vi "纳清蓝绿藻电极校准.vi"() -> ()   [LabVIEW 2016, in "斯坦道多参数.lvlib"]
uses:
  <vilib>/Utility/miscctls.llb/LVPointTypeDef.ctl
  <vilib>/Utility/miscctls.llb/LVPositionTypeDef.ctl
  <vilib>/Analysis/NI_AALBase.lvlib
panel:
  out "通讯状态":string
  out "温度校准参数":sgl
  out "第三点校准值":dbl
  out "标液3":sgl
  out "第二点校准值":dbl
  out "第一点校准值":dbl
  in  "校准停止":bool
  in  "校准启动":bool
  in  "校准模式":enum16{"两点校准", "单点校准", "三点校准"}(ring)=enum."单点校准"
  out "最小值":sgl format="%#.2f"
  out "最大值":sgl format="%#.2f"
  out "波形图表":u16(graph) caption="历史曲线"
  out "mean":dbl caption="均值" format="%#.2f"
  out "standard deviation":dbl caption="标准差" format="%#.2f"
  out "变异系数":dbl format="%#.6f"
  out "测量值":sgl
  out "提示":string
  out "标液2":sgl
  out "标液1":sgl
  out "原始光强数值":u16 caption="信号值"
  out "温度":dbl
  # "藻密度电极设定"
  # "℃"
  # "ug/L"
  # "℃"
  # "请选择校准模式:"
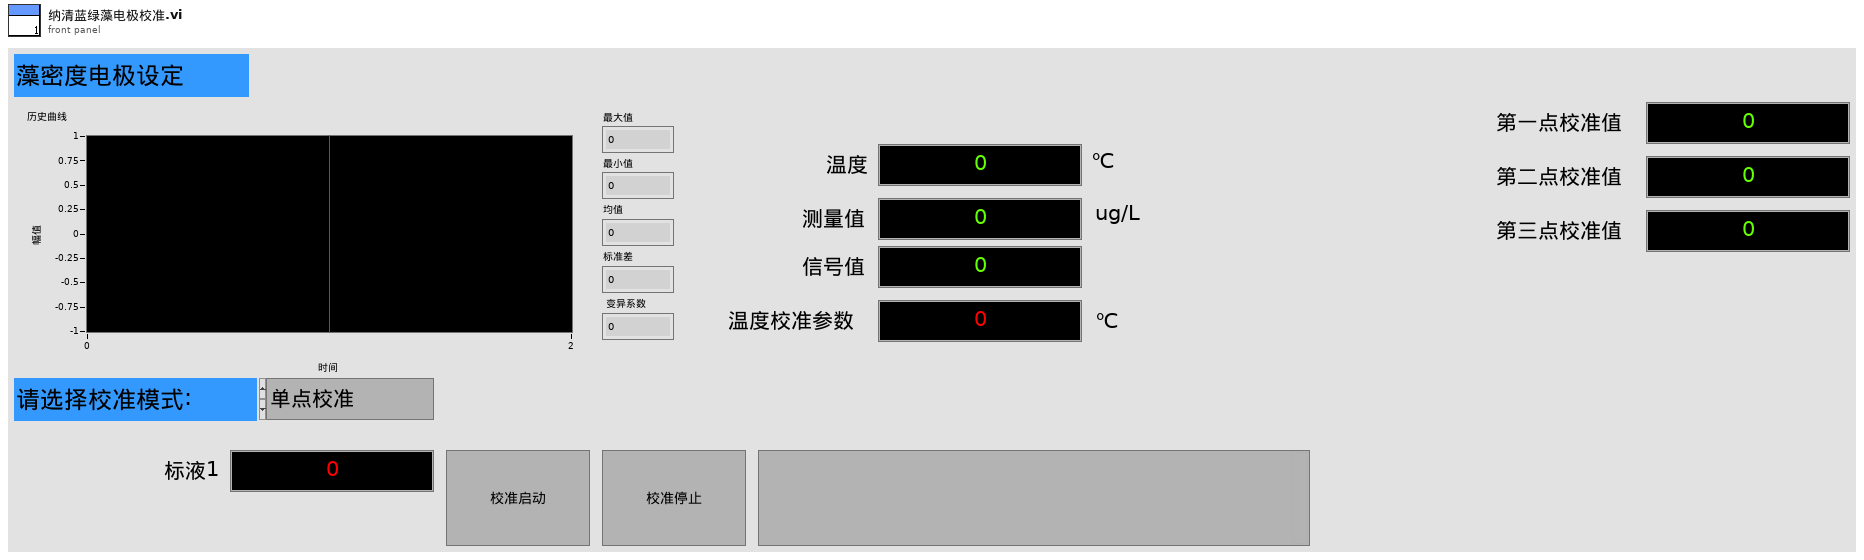
[diagram p1: front panel]
types:
  T1 = typedef "LVPointTypeDef.ctl" = cluster{"Horizontal":i16, "Vertical":i16}
  T2 = typedef "斯坦道多参数.lvlib/校准步骤.ctl" = enum16{"待机", "放置第一点标液", "第一点校准启动", "第一点校准写入", "第一点校准失败", "放置第二点标液", "第二点校准启动", "第二点校准写入", "第二点校准失败", "放置第三点标液", "第三点校准启动", "第三点校准写入", "第三点校准失败", "校准结果写入", "校准结束"}
  T3 = cluster{"报警码":u16, "蓝绿藻":sgl, "温度数据":sgl, "原始光强数值":u16, "0X0006_NC":u16, "平均次数":u16, "清扫模式":u16, "清扫次数":u16, "清扫间隔分钟":u16, "0X000B_NC":string, "产品名称":string, "序列号":string, "硬件版本":string, "软件版本":string, "通讯地址":u16, "波特率":u16, "设备类型":u16, "0X0026_NC":string, "0X0030_NC":u16, "第一点原始光强":u16, "第一点校准数据":sgl, "第二点原始光强":u16, "第二点校准数据":sgl, "第三点原始光强":u16, "第三点校准数据":sgl, "探头校准命令":u16, "温度校准参数":sgl, "温度校准命令":u16}
  T4 = typedef "LVPositionTypeDef.ctl" = cluster{"Left":i32, "Top":i32}
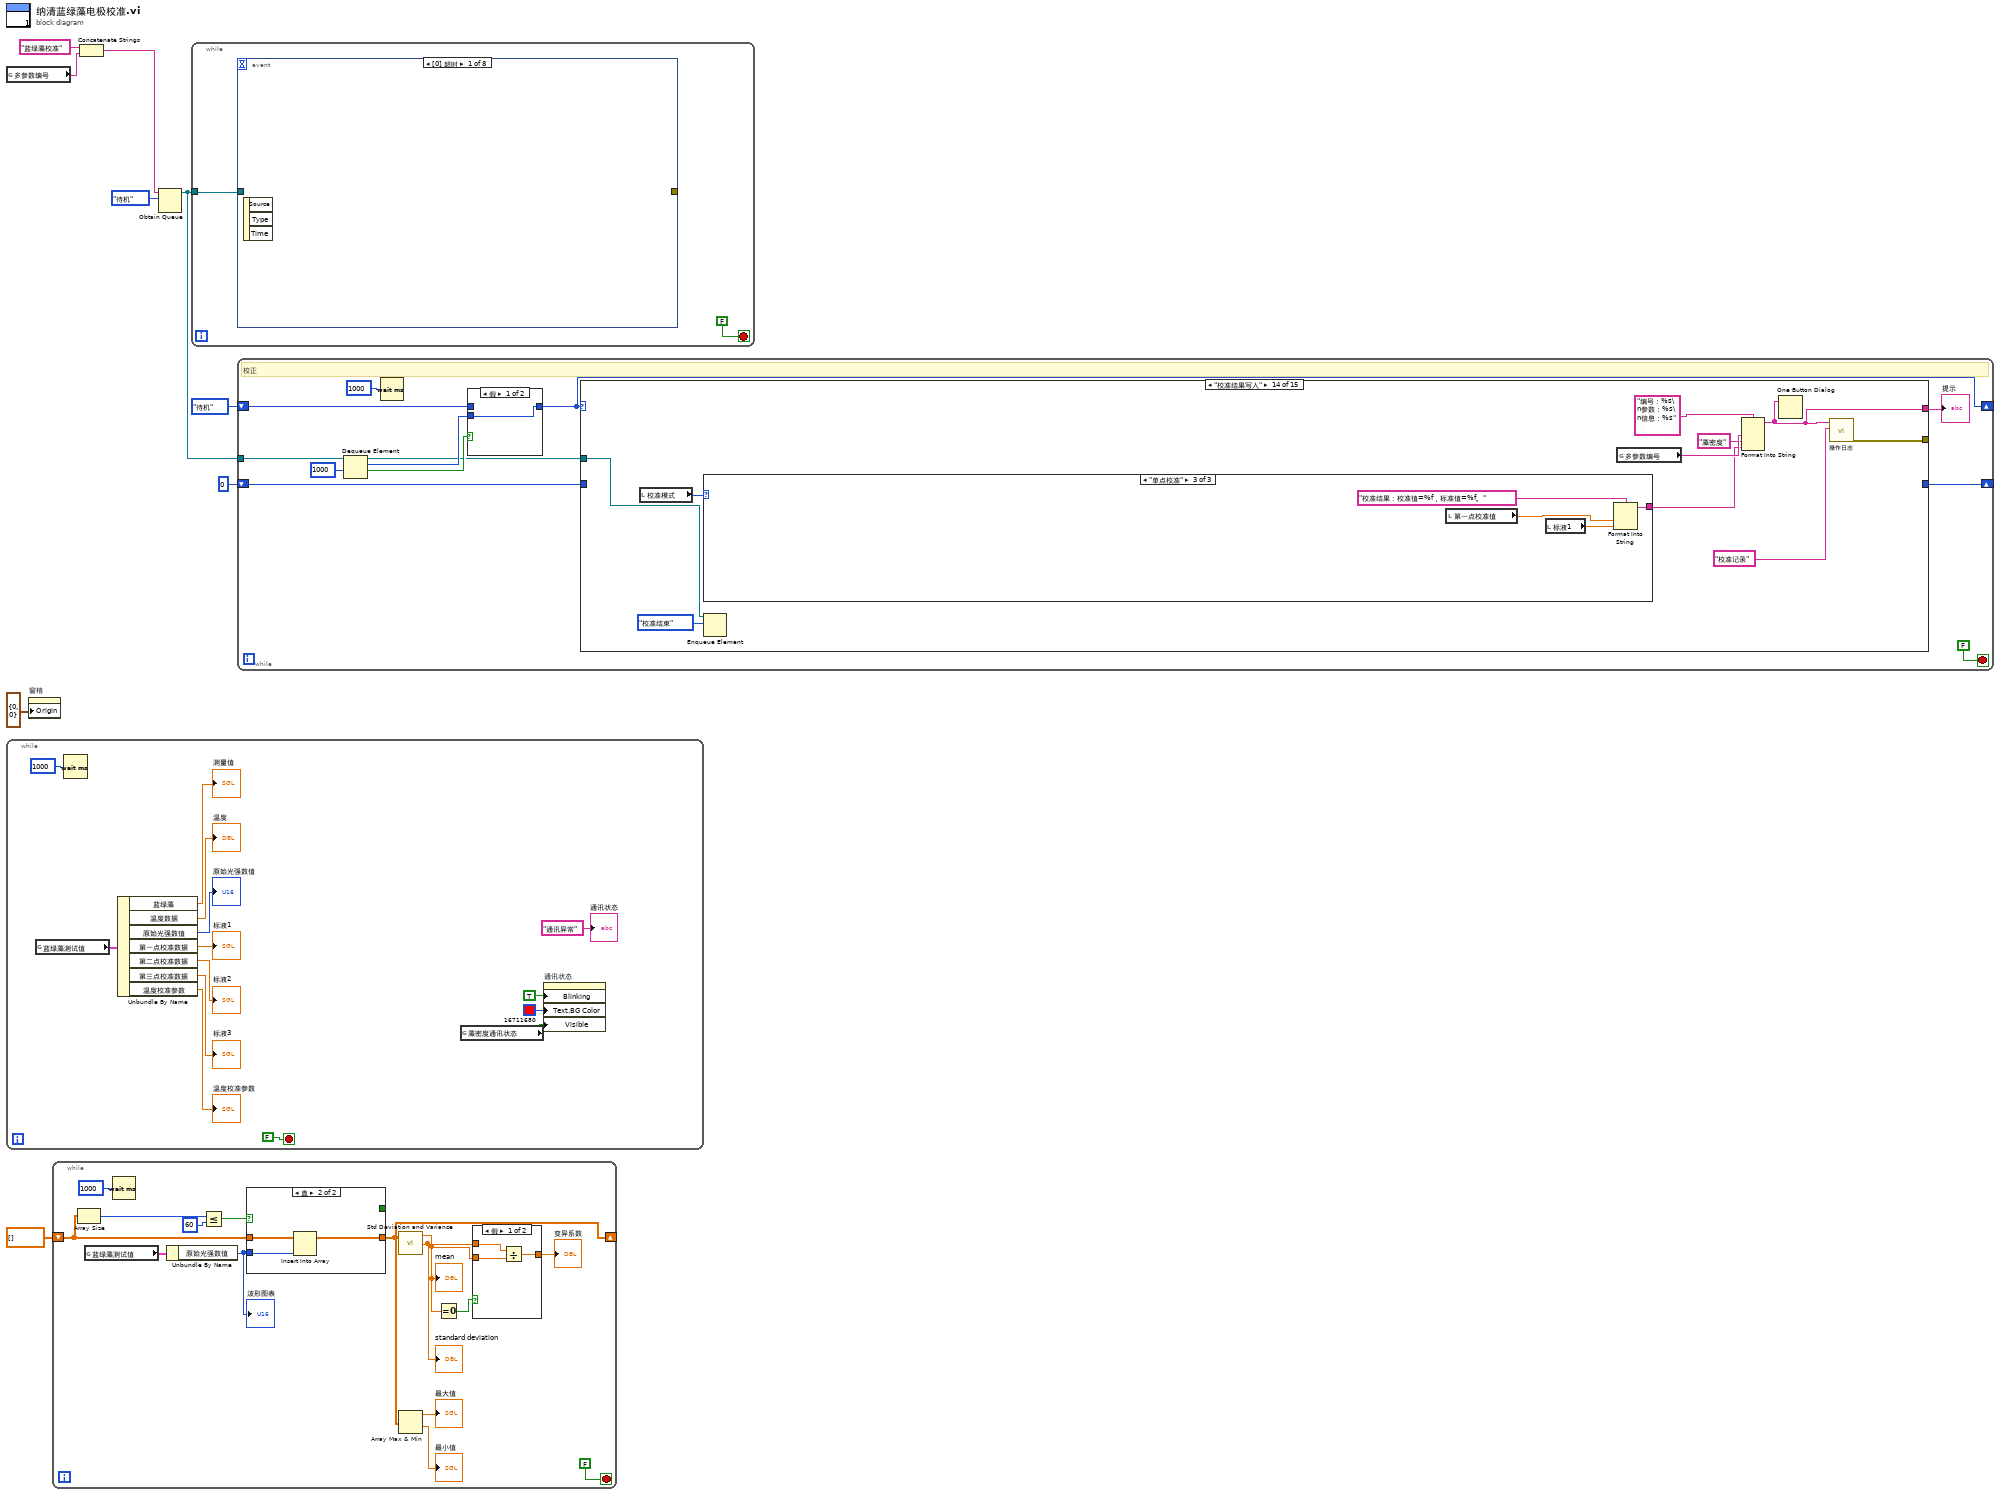
[diagram p0: block diagram]
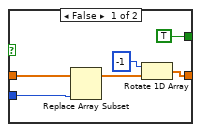
[diagram p3: hidden frame]
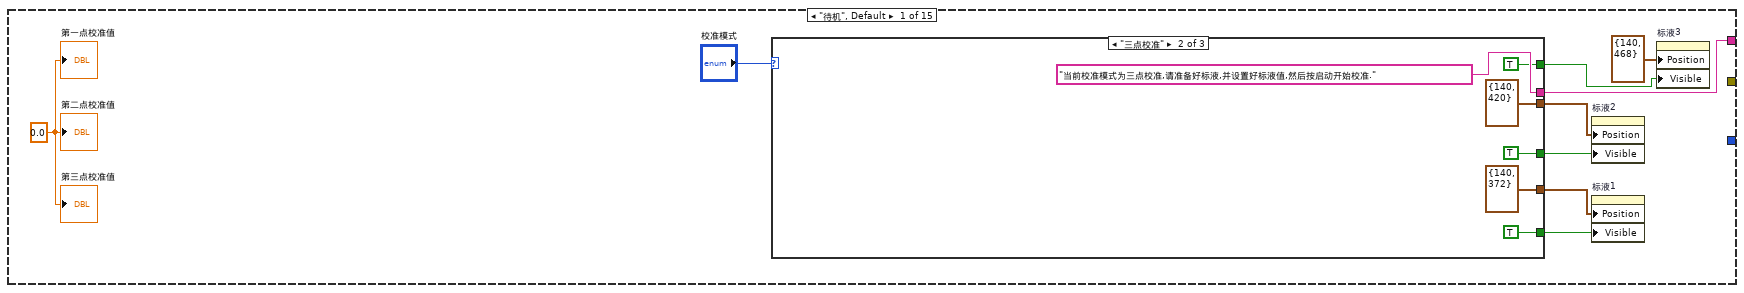
[diagram p5: hidden frame]
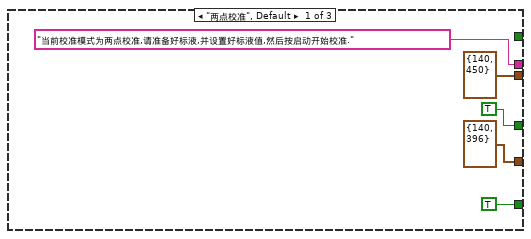
[diagram p6: hidden frame]
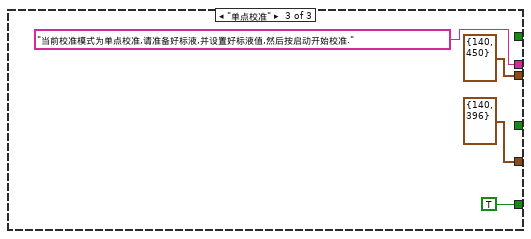
[diagram p7: hidden frame]
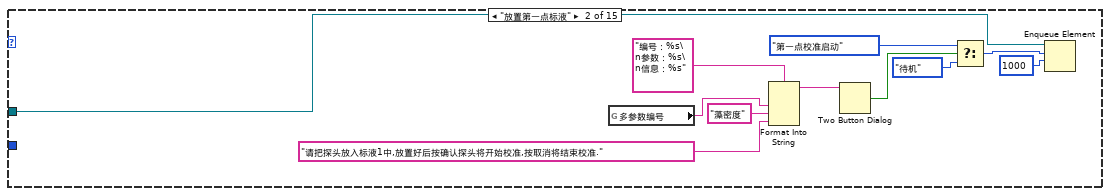
[diagram p8: hidden frame]
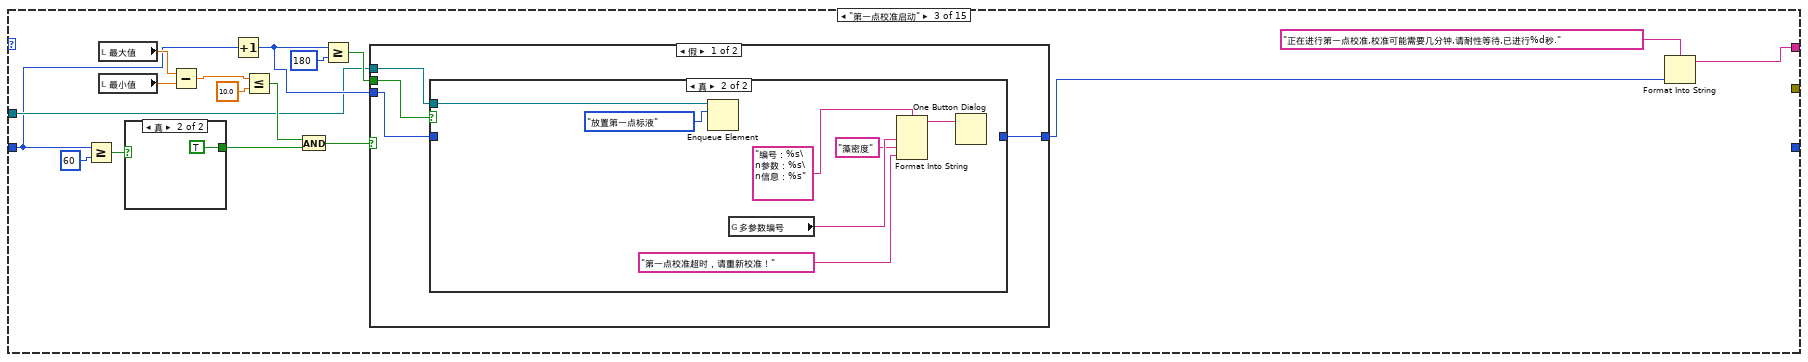
[diagram p9: hidden frame]
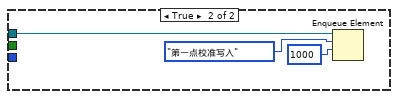
[diagram p11: hidden frame]
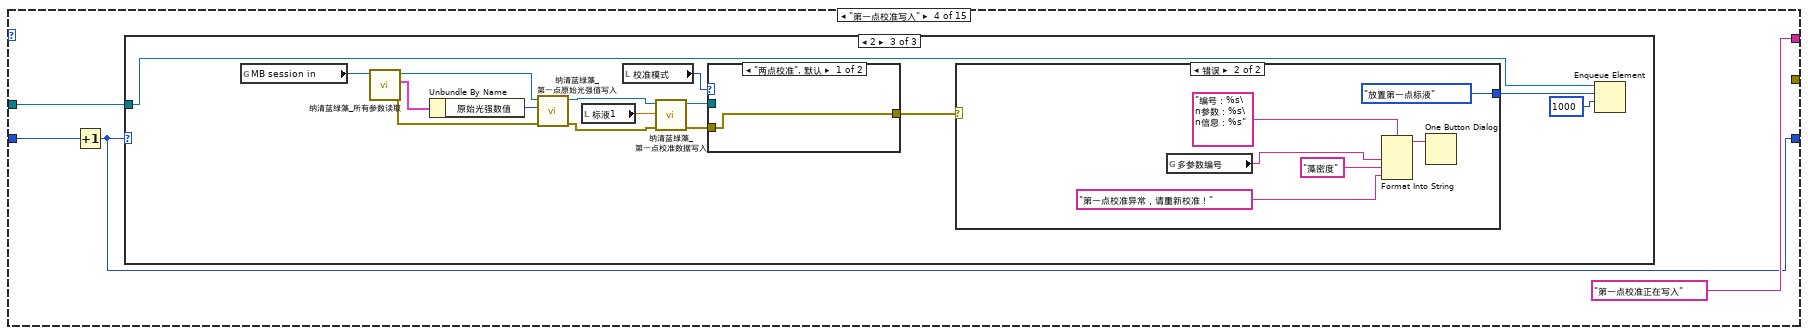
[diagram p13: hidden frame]
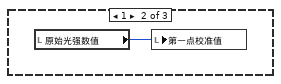
[diagram p15: hidden frame]
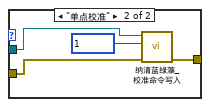
[diagram p16: hidden frame]
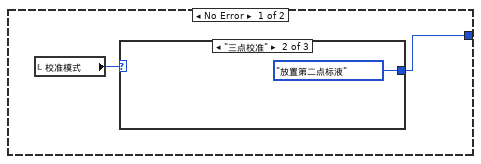
[diagram p17: hidden frame]
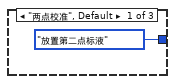
[diagram p18: hidden frame]
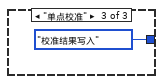
[diagram p19: hidden frame]
diagram:
  n1 = global read "多参数全局变量.vi" "多参数编号"() -> (w1:string)
  n2 = while {
    stop <- FALSE stop-if-true
    n3 = global read "纳清过程全局变量.vi" "蓝绿藻测试值"() -> (w21:T3)
    n4 = Wait (ms)(milliseconds to wait=u32 1000 ("等待时间（毫秒）")) -> ()  [unwired: 1 out]
    n5 = Unbundle By Name(w21) -> ("蓝绿藻"=→"测量值":sgl, "温度数据"=→"温度":sgl, "原始光强数值"=→"原始光强数值":u16, "第一点校准数据"=→"标液1":sgl, "第二点校准数据"=→"标液2":sgl, "第三点校准数据"=→"标液3":sgl, "温度校准参数"=→"温度校准参数":sgl)
    n6 = global read "多参数全局变量.vi" "藻密度通讯状态"() -> (w10:bool)
    n7 = property on="通讯状态" class="Str"("Blinking"=TRUE ("闪烁"), "Text.BG Color"=u32 16711680, "Visible"=w10) -> ()  [unwired: 2 in, 2 out]
    "通讯状态" <- "通讯异常" ("当前串口")
  }
  n8 = property on="窗格" class="Pane"("Origin"=T1 {"Horizontal"=0, "Vertical"=0} ("原点")) -> ()  [unwired: 2 in, 2 out]
  n9 = while {
    shift-right: [w28] -> _
    shift-left: sgl[] [] -> [w34]
    stop <- FALSE stop-if-true
    n10 = Array Size(array=w34) -> (size(s)=w36:i32)
    n11 = global read "纳清过程全局变量.vi" "蓝绿藻测试值"() -> (w24:T3)
    n12 = Wait (ms)(milliseconds to wait=u32 1000 ("等待时间（毫秒）")) -> ()  [unwired: 1 out]
    n13 = Unbundle By Name(w24) -> ("原始光强数值"=w25:u16)
    "波形图表" <- w25
    n14 = Less Or Equal?(x=w36, y=60) -> (x <= y?=w35:bool)
    n15 = case shown="真" w35 {
      tunnel: w34 -> [w47 w50]
      tunnel: w25 -> [w45 w49]
      tunnel: [w43 w48] -> w28
      tunnel: [TRUE _] -> _
      frame False {
        n16 = Replace Array Subset(array=w47, new element=w45) -> (w46:sgl[])  [unwired: 1 in]
        n17 = Rotate 1D Array(1:w46, 2:-1 ("n")) -> (0:w43:sgl[])
      }
      frame True {
        n18 = Insert Into Array(array=w50, new element=w49) -> (w48:sgl[])  [unwired: 1 in]
      }
    }
    n19 = call <vilib>:"Std Deviation and Variance.vi"("X"=w28) -> ("mean"=w32:dbl, "standard deviation"=w31:dbl)  [unwired: 1 in, 1 out]
    "mean" <- w32
    "standard deviation" <- w31
    n20 = Array Max & Min(array=w28) -> (max value=→"最大值":sgl, min value=→"最小值":sgl)  [unwired: 2 out]
    n21 = Equal To 0?(x=w32) -> (x = 0?=w33:bool)
    n22 = case shown="假" w33 {
      tunnel: w31 -> [w41 _]
      tunnel: [w40 _] -> w30
      tunnel: w32 -> [w39 _]
      frame False {
        n23 = Divide(x=w41, y=w39) -> (x/y=w40:dbl)
      }
      frame True {
      }
    }
    "变异系数" <- w30
  }
  n24 = Concatenate Strings("蓝绿藻校准" ("名称（未命名）"), w1) -> (w2:string)
  n25 = Obtain Queue(name (unnamed)=w2, element data type=校准步骤."待机" ("枚举")) -> (queue out=w4:refnum<queue>)  [unwired: 3 in, 2 out]
  n26 = while {
    tunnel: w4 -> [w51]
    stop <- FALSE stop-if-true
    n27 = event shown="[0] 超时" {
      selector: _ -> [_ _ _ _ _ _ _ _]
      dyn-events: _ -> [_ _ _ _ _ _ _ _]
      timeout: _ -> [_ _ _ _ _ _ _ _]
      tunnel: [_ _ w58 w62 w65 w66 _ _] -> _
      tunnel: w51 -> [_ _ _ _ _ _ w73 w75]
      event Timeout {
        n28 = event-data() -> ()  [unwired: 1 in, 3 out]
      }
      event "标液1", "标液2", "标液3", "温度校准参数": Mouse Down {
        n29 = event-data() -> ("CtlRef"=w53:refnum<vi>)  [unwired: 1 in, 7 out]
        n30 = property class="DigNum (严格)"(reference=w53) -> (reference out=w54:refnum<vi>, "Value"=w55:sgl)  [unwired: 1 in, 1 out]
        n31 = call "数字键盘.vi"("OldNumber"=w55) -> ("NewNumber"=w56:dbl)  [unwired: 1 in]
        n32 = property class="DigNum (严格)"(reference=w54, "Val(Sgnl)"=w56) -> ()  [unwired: 1 in, 2 out]
      }
      event "标液1": Value Change {
        n33 = event-data() -> ("NewVal"=w57:sgl)  [unwired: 1 in, 5 out]
        n34 = global read "多参数全局变量.vi" "MB session in"() -> (w59:refnum<class "MB_Master.lvclass">)
        n35 = call "纳清蓝绿藻_第一点校准数据写入.vi"("数值"=w57, "MB session in"=w59) -> ("error out"=w58:errorcluster)  [unwired: 8 in, 1 out]
      }
      event "标液2": Value Change {
        n36 = event-data() -> ("NewVal"=w61:sgl)  [unwired: 1 in, 5 out]
        n37 = global read "多参数全局变量.vi" "MB session in"() -> (w60:refnum<class "MB_Master.lvclass">)
        n38 = call "纳清蓝绿藻_第二点校准数据写入.vi"("数值"=w61, "MB session in"=w60) -> ("error out"=w62:errorcluster)  [unwired: 8 in, 1 out]
      }
      event "标液3": Value Change {
        n39 = event-data() -> ("NewVal"=w63:sgl)  [unwired: 1 in, 5 out]
        n40 = global read "多参数全局变量.vi" "MB session in"() -> (w64:refnum<class "MB_Master.lvclass">)
        n41 = call "纳清蓝绿藻_第三点校准数据写入.vi"("数值"=w63, "MB session in"=w64) -> ("error out"=w65:errorcluster)  [unwired: 8 in, 1 out]
      }
      event "温度校准参数": Value Change {
        n42 = event-data() -> ("NewVal"=w71:sgl)  [unwired: 1 in, 5 out]
        n43 = global read "多参数全局变量.vi" "MB session in"() -> (w70:refnum<class "MB_Master.lvclass">)
        n44 = call "纳清蓝绿藻_温度校准参数写入.vi"("数值"=w71, "MB session in"=w70) -> ("error out"=w72:errorcluster, "MB session out"=w69:refnum<class "MB_Master.lvclass">)  [unwired: 8 in]
        n45 = call "纳清蓝绿藻_温度校准命令写入.vi"("error in (no error)"=w72, "数值"=u16 1 ("starting address"), "MB session in"=w69) -> ("error out"=w67:errorcluster)  [unwired: 7 in, 1 out]
        n46 = call <vilib>:"Simple Error Handler.vi"("error in (no error)"=w67) -> ("error out"=w66:errorcluster)  [unwired: 4 in, 4 out]
      }
      event "校准启动": Value Change {
        n47 = event-data() -> ()  [unwired: 1 in, 6 out]
        n48 = Enqueue Element(queue=w73, element=校准步骤."放置第一点标液" ("元素")) -> ()  [unwired: 2 in, 3 out]
      }
      event "校准停止": Value Change {
        n49 = event-data() -> ()  [unwired: 1 in, 6 out]
        n50 = Flush Queue(queue=w75) -> (queue out=w76:refnum<queue>)  [unwired: 1 in, 2 out]
        n51 = Enqueue Element(queue=w76, element=校准步骤."待机" ("元素"), timeout in ms (-1)=1000 ("超时毫秒(-1)")) -> ()  [unwired: 1 in, 3 out]
      }
    }
  }
  n52 = while "While循环" {
    shift-right: [w80] -> _
    shift-left: 校准步骤."待机" ("枚举") -> [w82]
    shift-right: [w79] -> _
    shift-left: 0 -> [w88]
    tunnel: w4 -> [w83]
    stop <- FALSE stop-if-true
    # "校正"
    n53 = Dequeue Element(queue=w83, timeout in ms (-1)=1000 ("超时毫秒(-1)")) -> (queue out=w81:refnum<queue>, element=w84:T2, timed out?=w85:bool)  [unwired: 1 in, 1 out]
    n54 = Wait (ms)(milliseconds to wait=u32 1000 ("等待时间（毫秒）")) -> ()  [unwired: 1 out]
    n55 = case shown="假" w85 {
      tunnel: w84 -> [w91 _]
      tunnel: [w91 w92] -> w80
      tunnel: w82 -> [_ w92]
      frame False {
      }
      frame True {
      }
    }
    n56 = case shown="\"校准结果写入\"" w80 {
      tunnel: [w100 _ w128 "第一点校准正在写入" ("提示") _ _ w210 "第二点校准正在写入" ("提示") "第二点校准失败" ("提示") _ "第三点校准正在写入" ("提示") w322 "第三点校准失败" ("提示") w355 w382] -> w87
      tunnel: w88 -> [_ _ w130 w163 _ _ w211 w243 _ _ w291 w323 _ _ _]
      tunnel: [_ _ _ w161 _ _ w209 w241 _ _ w289 w321 _ _ _] -> w79
      tunnel: w81 -> [_ w123 w131 w162 _ w202 w212 w242 _ w283 w290 w324 _ w362 _]
      tunnel: [_ _ _ _ _ _ _ _ _ _ _ _ _ w360 _] -> _
      frame "待机", Default {
        w93 = 0.0 ("第一点校准值")
        n57 = case shown="\"三点校准\"" "校准模式" {
          tunnel: ["当前校准模式为两点校准,请准备好标液,并设置好标液值,然后按启动开始校准." ("提示") "当前校准模式为三点校准,请准备好标液,并设置好标液值,然后按启动开始校准." ("提示") "当前校准模式为单点校准,请准备好标液,并设置好标液值,然后按启动开始校准." ("提示")] -> w100
          tunnel: [TRUE ("可见") TRUE ("可见") _] -> w96
          tunnel: [T4 {"Left"=140, "Top"=396} ("位置") T4 {"Left"=140, "Top"=372} ("位置") T4 {"Left"=140, "Top"=396} ("位置")] -> w99
          tunnel: [T4 {"Left"=140, "Top"=450} ("位置 2") T4 {"Left"=140, "Top"=420} ("位置 2") T4 {"Left"=140, "Top"=450} ("位置 2")] -> w98
          tunnel: [_ TRUE ("可见") _] -> w95
          tunnel: [TRUE ("可见") TRUE ("可见") TRUE ("可见")] -> w94
          frame "两点校准", Default {
          }
          frame "三点校准" {
          }
          frame "单点校准" {
          }
        }
        n58 = property on="标液2" class="DigNum (严格)"("Position"=w98, "Visible"=w96) -> ()  [unwired: 2 in, 2 out]
        n59 = property on="标液1" class="DigNum (严格)"("Position"=w99, "Visible"=w94) -> ()  [unwired: 2 in, 2 out]
        n60 = property on="标液3" class="DigNum (严格)"("Position"=T4 {"Left"=140, "Top"=468} ("位置 3"), "Visible"=w95) -> ()  [unwired: 2 in, 2 out]
        "第一点校准值" <- w93
        "第二点校准值" <- w93
        "第三点校准值" <- w93
      }
      frame "放置第一点标液" {
        n61 = global read "多参数全局变量.vi" "多参数编号"() -> (w121:string)
        n62 = Format Into String(format string="编号：%s\n参数：%s\n信息：%s" ("格式字符串"), w121, "藻密度" ("输入 2"), "请把探头放入标液1中,放置好后按确认探头将开始校准,按取消将结束校准." ("消息")) -> (resulting string=w119:string)  [unwired: 2 in, 1 out]
        n63 = Two Button Dialog(message=w119) -> (T button?=w117:bool)  [unwired: 2 in]
        n64 = Select(t=校准步骤."第一点校准启动" ("元素"), s=w117, f=校准步骤."待机" ("元素")) -> (s? t:f=w124:T2)
        n65 = Enqueue Element(queue=w123, element=w124, timeout in ms (-1)=1000 ("超时毫秒(-1)")) -> ()  [unwired: 1 in, 3 out]
      }
      frame "第一点校准启动" {
        n66 = Greater Or Equal?(x=w130, y=60) -> (x >= y?=w137:bool)
        n67 = local read "最大值"() -> (w140:sgl)
        n68 = local read "最小值"() -> (w139:sgl)
        n69 = case shown="真" w137 {
          tunnel: [_ TRUE] -> w138
          frame False {
          }
          frame True {
          }
        }
        n70 = Subtract(x=w140, y=w139) -> (x-y=w141:sgl)
        n71 = Increment(x=w130) -> (x+1=w144:i32)
        n72 = Less Or Equal?(x=w141, y=10.0) -> (x <= y?=w134:bool)
        n73 = And(x=w134, y=w138) -> (x .and. y?=w142:bool)
        n74 = Greater Or Equal?(x=w144, y=180) -> (x >= y?=w143:bool)
        n75 = case shown="假" w142 {
          tunnel: w131 -> [w147 w159]
          tunnel: w143 -> [w148 _]
          tunnel: w144 -> [w146 _]
          tunnel: [w145 _] -> w129
          frame False {
            n76 = case shown="真" w148 {
              tunnel: w147 -> [_ w156]
              tunnel: w146 -> [w149 _]
              tunnel: [w149 _] -> w145
              frame False {
              }
              frame True {
                n77 = Enqueue Element(queue=w156, element=校准步骤."放置第一点标液" ("元素")) -> ()  [unwired: 2 in, 3 out]
                n78 = global read "多参数全局变量.vi" "多参数编号"() -> (w153:string)
                n79 = Format Into String(format string="编号：%s\n参数：%s\n信息：%s" ("格式字符串"), w153, "藻密度" ("输入 2"), "第一点校准超时，请重新校准！" ("error source (\" \")")) -> (resulting string=w150:string)  [unwired: 2 in, 1 out]
                n80 = One Button Dialog(message=w150) -> ()  [unwired: 1 in, 1 out]
              }
            }
          }
          frame True {
            n81 = Enqueue Element(queue=w159, element=校准步骤."第一点校准写入" ("元素"), timeout in ms (-1)=1000 ("超时毫秒(-1)")) -> ()  [unwired: 1 in, 3 out]
          }
        }
        n82 = Format Into String(format string="正在进行第一点校准,校准可能需要几分钟,请耐性等待,已进行%d秒." ("格式字符串"), w129) -> (resulting string=w128:string)  [unwired: 2 in, 1 out]
      }
      frame "第一点校准写入" {
        n83 = Increment(x=w163) -> (x+1=w161:i32)
        n84 = case shown="2" w161 {
          tunnel: w162 -> [_ _ w180]
          frame 0, Default {
          }
          frame 1 {
            n85 = local read "原始光强数值"() -> (w165:u16)
            n86 = local write "第一点校准值"(w165) -> ()
          }
          frame 2 {
            n87 = global read "多参数全局变量.vi" "MB session in"() -> (w176:refnum<class "MB_Master.lvclass">)
            n88 = call "纳清蓝绿藻_所有参数读取.vi"("MB session in"=w176) -> ("error out"=w178:errorcluster, "输出值"=w175:T3, "MB session out"=w177:refnum<class "MB_Master.lvclass">)  [unwired: 8 in]
            n89 = Unbundle By Name(w175) -> ("原始光强数值"=w174:u16)
            n90 = call "纳清蓝绿藻_第一点原始光强值写入.vi"("error in (no error)"=w178, "数值"=w174, "MB session in"=w177) -> ("error out"=w173:errorcluster, "MB session out"=w172:refnum<class "MB_Master.lvclass">)  [unwired: 7 in]
            n91 = local read "标液1"() -> (w169:sgl)
            n92 = local read "校准模式"() -> (w166:enum16{"两点校准", "单点校准", "三点校准"})
            n93 = call "纳清蓝绿藻_第一点校准数据写入.vi"("error in (no error)"=w173, "数值"=w169, "MB session in"=w172) -> ("error out"=w171:errorcluster, "MB session out"=w170:refnum<class "MB_Master.lvclass">)  [unwired: 7 in]
            n94 = case shown="\"两点校准\", 默认" w166 {
              tunnel: w171 -> [w181 w185]
              tunnel: w170 -> [_ w184]
              tunnel: [w181 w182] -> w168
              frame "两点校准", Default {
              }
              frame "单点校准" {
                n95 = call "纳清蓝绿藻_校准命令写入.vi"("error in (no error)"=w185, "数值"=u16 1 ("starting address"), "MB session in"=w184) -> ("error out"=w182:errorcluster)  [unwired: 7 in, 1 out]
              }
            }
            n96 = case shown="错误" w168 {
              tunnel: [w186 校准步骤."放置第一点标液" ("元素")] -> w167
              frame No Error {
                n97 = local read "校准模式"() -> (w187:enum16{"两点校准", "单点校准", "三点校准"})
                n98 = case shown="\"三点校准\"" w187 {
                  tunnel: [校准步骤."放置第二点标液" ("元素") 校准步骤."放置第二点标液" ("元素") 校准步骤."校准结果写入" ("元素")] -> w186
                  frame "两点校准", Default {
                  }
                  frame "三点校准" {
                  }
                  frame "单点校准" {
                  }
                }
              }
              frame Error {
                n99 = global read "多参数全局变量.vi" "多参数编号"() -> (w195:string)
                n100 = Format Into String(format string="编号：%s\n参数：%s\n信息：%s" ("格式字符串"), w195, "藻密度" ("输入 2"), "第一点校准异常，请重新校准！" ("error source (\" \")")) -> (resulting string=w192:string)  [unwired: 2 in, 1 out]
                n101 = One Button Dialog(message=w192) -> ()  [unwired: 1 in, 1 out]
              }
            }
            n102 = Enqueue Element(queue=w180, element=w167, timeout in ms (-1)=1000 ("超时毫秒(-1)")) -> ()  [unwired: 1 in, 3 out]
          }
        }
      }
      frame "第一点校准失败" {
      }
      frame "放置第二点标液" {
        n103 = global read "多参数全局变量.vi" "多参数编号"() -> (w200:string)
        n104 = Format Into String(format string="编号：%s\n参数：%s\n信息：%s" ("格式字符串"), w200, "藻密度" ("输入 2"), "请把探头放入标液2中,放置好后按确认将继续校准,按取消将结束校准." ("消息")) -> (resulting string=w198:string)  [unwired: 2 in, 1 out]
        n105 = Two Button Dialog(message=w198) -> (T button?=w206:bool)  [unwired: 2 in]
        n106 = Select(t=校准步骤."第二点校准启动" ("元素"), s=w206, f=校准步骤."待机" ("元素")) -> (s? t:f=w203:T2)
        n107 = Enqueue Element(queue=w202, element=w203, timeout in ms (-1)=1000 ("超时毫秒(-1)")) -> ()  [unwired: 1 in, 3 out]
      }
      frame "第二点校准启动" {
        n108 = Greater Or Equal?(x=w211, y=60) -> (x >= y?=w217:bool)
        n109 = local read "最大值"() -> (w220:sgl)
        n110 = local read "最小值"() -> (w219:sgl)
        n111 = case shown="真" w217 {
          tunnel: [_ TRUE] -> w218
          frame False {
          }
          frame True {
          }
        }
        n112 = Subtract(x=w220, y=w219) -> (x-y=w221:sgl)
        n113 = Increment(x=w211) -> (x+1=w224:i32)
        n114 = Less Or Equal?(x=w221, y=10.0) -> (x <= y?=w214:bool)
        n115 = And(x=w214, y=w218) -> (x .and. y?=w222:bool)
        n116 = Greater Or Equal?(x=w224, y=180) -> (x >= y?=w223:bool)
        n117 = case shown="假" w222 {
          tunnel: w212 -> [w227 w239]
          tunnel: w223 -> [w228 _]
          tunnel: w224 -> [w226 _]
          tunnel: [w225 _] -> w209
          frame False {
            n118 = case shown="真" w228 {
              tunnel: w227 -> [_ w236]
              tunnel: w226 -> [w229 _]
              tunnel: [w229 _] -> w225
              frame False {
              }
              frame True {
                n119 = Enqueue Element(queue=w236, element=校准步骤."放置第二点标液" ("元素")) -> ()  [unwired: 2 in, 3 out]
                n120 = global read "多参数全局变量.vi" "多参数编号"() -> (w233:string)
                n121 = Format Into String(format string="编号：%s\n参数：%s\n信息：%s" ("格式字符串"), w233, "藻密度" ("输入 2"), "第二点校准超时，请重新校准！" ("消息")) -> (resulting string=w231:string)  [unwired: 2 in, 1 out]
                n122 = One Button Dialog(message=w231) -> ()  [unwired: 1 in, 1 out]
              }
            }
          }
          frame True {
            n123 = Enqueue Element(queue=w239, element=校准步骤."第二点校准写入" ("元素"), timeout in ms (-1)=1000 ("超时毫秒(-1)")) -> ()  [unwired: 1 in, 3 out]
          }
        }
        n124 = Format Into String(format string="正在进行第二点校准,校准可能需要几分钟,请耐性等待,已进行%d秒." ("格式字符串"), w209) -> (resulting string=w210:string)  [unwired: 2 in, 1 out]
      }
      frame "第二点校准写入" {
        n125 = Increment(x=w243) -> (x+1=w241:i32)
        n126 = case shown="2" w241 {
          tunnel: w242 -> [_ _ w260]
          frame 0, Default {
          }
          frame 1 {
            n127 = local read "原始光强数值"() -> (w245:u16)
            n128 = local write "第二点校准值"(w245) -> ()
          }
          frame 2 {
            n129 = global read "多参数全局变量.vi" "MB session in"() -> (w256:refnum<class "MB_Master.lvclass">)
            n130 = call "纳清蓝绿藻_所有参数读取.vi"("MB session in"=w256) -> ("error out"=w258:errorcluster, "输出值"=w255:T3, "MB session out"=w257:refnum<class "MB_Master.lvclass">)  [unwired: 8 in]
            n131 = Unbundle By Name(w255) -> ("原始光强数值"=w254:u16)
            n132 = call "纳清蓝绿藻_第二点原始光强值写入.vi"("error in (no error)"=w258, "数值"=w254, "MB session in"=w257) -> ("error out"=w253:errorcluster, "MB session out"=w252:refnum<class "MB_Master.lvclass">)  [unwired: 7 in]
            n133 = local read "标液2"() -> (w249:sgl)
            n134 = local read "校准模式"() -> (w246:enum16{"两点校准", "单点校准", "三点校准"})
            n135 = call "纳清蓝绿藻_第二点校准数据写入.vi"("error in (no error)"=w253, "数值"=w249, "MB session in"=w252) -> ("error out"=w251:errorcluster, "MB session out"=w250:refnum<class "MB_Master.lvclass">)  [unwired: 7 in]
            n136 = case shown="\"两点校准\"" w246 {
              tunnel: w251 -> [w264 w265]
              tunnel: w250 -> [w263 _]
              tunnel: [w261 w265] -> w248
              frame "两点校准" {
                n137 = call "纳清蓝绿藻_校准命令写入.vi"("error in (no error)"=w264, "数值"=u16 2 ("starting address"), "MB session in"=w263) -> ("error out"=w261:errorcluster)  [unwired: 7 in, 1 out]
              }
              frame "单点校准", Default {
              }
            }
            n138 = case shown="错误" w248 {
              tunnel: [w266 校准步骤."放置第二点标液" ("元素")] -> w247
              frame No Error {
                n139 = local read "校准模式"() -> (w267:enum16{"两点校准", "单点校准", "三点校准"})
                n140 = case shown="\"单点校准\"" w267 {
                  tunnel: [校准步骤."校准结果写入" ("元素") 校准步骤."放置第三点标液" ("元素") 校准步骤."校准结果写入" ("元素")] -> w266
                  frame "两点校准", Default {
                  }
                  frame "三点校准" {
                  }
                  frame "单点校准" {
                  }
                }
              }
              frame Error {
                n141 = global read "多参数全局变量.vi" "多参数编号"() -> (w275:string)
                n142 = Format Into String(format string="编号：%s\n参数：%s\n信息：%s" ("格式字符串"), w275, "藻密度" ("输入 2"), "第二点校准异常，请重新校准！" ("error source (\" \")")) -> (resulting string=w272:string)  [unwired: 2 in, 1 out]
                n143 = One Button Dialog(message=w272) -> ()  [unwired: 1 in, 1 out]
              }
            }
            n144 = Enqueue Element(queue=w260, element=w247, timeout in ms (-1)=1000 ("超时毫秒(-1)")) -> ()  [unwired: 1 in, 3 out]
          }
        }
      }
      frame "第二点校准失败" {
      }
      frame "放置第三点标液" {
        n145 = global read "多参数全局变量.vi" "多参数编号"() -> (w281:string)
        n146 = Format Into String(format string="编号：%s\n参数：%s\n信息：%s" ("格式字符串"), w281, "藻密度" ("输入 2"), "请把探头放入标液3中,放置好后按确认将继续校准,按取消将结束校准." ("消息")) -> (resulting string=w279:string)  [unwired: 2 in, 1 out]
        n147 = Two Button Dialog(message=w279) -> (T button?=w287:bool)  [unwired: 2 in]
        n148 = Select(t=校准步骤."第三点校准启动" ("元素"), s=w287, f=校准步骤."待机" ("元素")) -> (s? t:f=w284:T2)
        n149 = Enqueue Element(queue=w283, element=w284, timeout in ms (-1)=1000 ("超时毫秒(-1)")) -> ()  [unwired: 1 in, 3 out]
      }
      frame "第三点校准写入" {
        n150 = Increment(x=w291) -> (x+1=w289:i32)
        n151 = case shown="2" w289 {
          tunnel: w290 -> [_ _ w295]
          frame 0, Default {
          }
          frame 1 {
            n152 = local read "原始光强数值"() -> (w293:u16)
            n153 = local write "第二点校准值"(w293) -> ()
          }
          frame 2 {
            n154 = global read "多参数全局变量.vi" "MB session in"() -> (w306:refnum<class "MB_Master.lvclass">)
            n155 = call "纳清蓝绿藻_所有参数读取.vi"("MB session in"=w306) -> ("error out"=w308:errorcluster, "输出值"=w305:T3, "MB session out"=w307:refnum<class "MB_Master.lvclass">)  [unwired: 8 in]
            n156 = Unbundle By Name(w305) -> ("原始光强数值"=w304:u16)
            n157 = call "纳清蓝绿藻_第三点原始光强值写入.vi"("error in (no error)"=w308, "数值"=w304, "MB session in"=w307) -> ("error out"=w303:errorcluster, "MB session out"=w302:refnum<class "MB_Master.lvclass">)  [unwired: 7 in]
            n158 = local read "标液3"() -> (w298:sgl)
            n159 = call "纳清蓝绿藻_第三点校准数据写入.vi"("error in (no error)"=w303, "数值"=w298, "MB session in"=w302) -> ("error out"=w301:errorcluster, "MB session out"=w300:refnum<class "MB_Master.lvclass">)  [unwired: 7 in]
            n160 = call "纳清蓝绿藻_校准命令写入.vi"("error in (no error)"=w301, "数值"=u16 3 ("starting address"), "MB session in"=w300) -> ("error out"=w297:errorcluster)  [unwired: 7 in, 1 out]
            n161 = case shown="错误" w297 {
              tunnel: [w309 校准步骤."放置第三点标液" ("元素")] -> w294
              frame No Error {
                n162 = local read "校准模式"() -> (w310:enum16{"两点校准", "单点校准", "三点校准"})
                n163 = case shown="\"三点校准\"" w310 {
                  tunnel: [校准步骤."放置第二点标液" ("元素") 校准步骤."校准结果写入" ("元素") 校准步骤."校准结果写入" ("元素")] -> w309
                  frame "两点校准", Default {
                  }
                  frame "三点校准" {
                  }
                  frame "单点校准" {
                  }
                }
              }
              frame Error {
                n164 = global read "多参数全局变量.vi" "多参数编号"() -> (w318:string)
                n165 = Format Into String(format string="编号：%s\n参数：%s\n信息：%s" ("格式字符串"), w318, "藻密度" ("输入 2"), "第三点校准异常，请重新校准！" ("error source (\" \")")) -> (resulting string=w315:string)  [unwired: 2 in, 1 out]
                n166 = One Button Dialog(message=w315) -> ()  [unwired: 1 in, 1 out]
              }
            }
            n167 = Enqueue Element(queue=w295, element=w294, timeout in ms (-1)=1000 ("超时毫秒(-1)")) -> ()  [unwired: 1 in, 3 out]
          }
        }
      }
      frame "第三点校准启动" {
        n168 = Greater Or Equal?(x=w323, y=60) -> (x >= y?=w329:bool)
        n169 = local read "最大值"() -> (w332:sgl)
        n170 = local read "最小值"() -> (w331:sgl)
        n171 = case shown="真" w329 {
          tunnel: [_ TRUE] -> w330
          frame False {
          }
          frame True {
          }
        }
        n172 = Subtract(x=w332, y=w331) -> (x-y=w333:sgl)
        n173 = Increment(x=w323) -> (x+1=w336:i32)
        n174 = Less Or Equal?(x=w333, y=10.0) -> (x <= y?=w326:bool)
        n175 = And(x=w326, y=w330) -> (x .and. y?=w334:bool)
        n176 = Greater Or Equal?(x=w336, y=180) -> (x >= y?=w335:bool)
        n177 = case shown="假" w334 {
          tunnel: w324 -> [w339 w351]
          tunnel: w335 -> [w340 _]
          tunnel: w336 -> [w338 _]
          tunnel: [w337 _] -> w321
          frame False {
            n178 = case shown="真" w340 {
              tunnel: w339 -> [_ w348]
              tunnel: w338 -> [w341 _]
              tunnel: [w341 _] -> w337
              frame False {
              }
              frame True {
                n179 = Enqueue Element(queue=w348, element=校准步骤."放置第三点标液" ("元素")) -> ()  [unwired: 2 in, 3 out]
                n180 = global read "多参数全局变量.vi" "多参数编号"() -> (w345:string)
                n181 = Format Into String(format string="编号：%s\n参数：%s\n信息：%s" ("格式字符串"), w345, "藻密度" ("输入 2"), "第三点校准异常，请重新校准！" ("error source (\" \")")) -> (resulting string=w342:string)  [unwired: 2 in, 1 out]
                n182 = One Button Dialog(message=w342) -> ()  [unwired: 1 in, 1 out]
              }
            }
          }
          frame True {
            n183 = Enqueue Element(queue=w351, element=校准步骤."第三点校准写入" ("元素"), timeout in ms (-1)=1000 ("超时毫秒(-1)")) -> ()  [unwired: 1 in, 3 out]
          }
        }
        n184 = Format Into String(format string="正在进行第三点校准,校准可能需要几分钟,请耐性等待,已进行%d秒." ("格式字符串"), w321) -> (resulting string=w322:string)  [unwired: 2 in, 1 out]
      }
      frame "第三点校准失败" {
      }
      frame "校准结果写入" {
        n185 = local read "校准模式"() -> (w361:enum16{"两点校准", "单点校准", "三点校准"})
        n186 = case shown="\"单点校准\"" w361 {
          tunnel: [w366 w374 w381] -> w356
          frame "两点校准", Default {
            n187 = local read "第一点校准值"() -> (w369:dbl)
            n188 = local read "第二点校准值"() -> (w365:dbl)
            n189 = local read "标液1"() -> (w367:sgl)
            n190 = local read "标液2"() -> (w364:sgl)
            n191 = Format Into String(format string="校准结果：第一点校准值=%f，第一点标准值=%f,第二点校准值=%f，第二点标准值=%f." ("提示"), w369, w367, w365, w364) -> (resulting string=w366:string)  [unwired: 2 in, 1 out]
          }
          frame "三点校准" {
            n192 = local read "第一点校准值"() -> (w377:dbl)
            n193 = local read "第二点校准值"() -> (w373:dbl)
            n194 = local read "第三点校准值"() -> (w371:dbl)
            n195 = local read "标液1"() -> (w375:sgl)
            n196 = local read "标液2"() -> (w372:sgl)
            n197 = local read "标液3"() -> (w370:sgl)
            n198 = Format Into String(format string="校准结果：第一点校准值=%f，第一点标准值=%f,第二点校准值=%f，第二点标准值=%f,第三点校准值=%f，第三点标准值=%f." ("提示"), w377, w375, w373, w372, w371, w370) -> (resulting string=w374:string)  [unwired: 2 in, 1 out]
          }
          frame "单点校准" {
            n199 = local read "第一点校准值"() -> (w380:dbl)
            n200 = local read "标液1"() -> (w378:sgl)
            n201 = Format Into String(format string="校准结果：校准值=%f，标准值=%f。" ("提示"), w380, w378) -> (resulting string=w381:string)  [unwired: 2 in, 1 out]
          }
        }
        n202 = Enqueue Element(queue=w362, element=校准步骤."校准结束" ("元素")) -> ()  [unwired: 2 in, 3 out]
        n203 = global read "多参数全局变量.vi" "多参数编号"() -> (w358:string)
        n204 = Format Into String(format string="编号：%s\n参数：%s\n信息：%s" ("格式字符串"), w358, "藻密度" ("输入 2"), w356) -> (resulting string=w355:string)  [unwired: 2 in, 1 out]
        n205 = One Button Dialog(message=w355) -> ()  [unwired: 1 in, 1 out]
        n206 = call "操作日志.vi"("table"="校准记录", "日志信息"=w355) -> ("error out"=w360:errorcluster)  [unwired: 9 in]
      }
      frame "校准结束" {
        n207 = local read "提示"() -> (w382:string)
      }
    }
    "提示" <- w87
  }
